vi "Charging_Wait for Charge State.vi"(6 "2nd expected ChargingState (NaN)":string="NaN", 7 "expected ChargingState":string="CHARGE_CC_SLOW-3", 8 "error in":errorcluster, 9 "Abort Threshold (42 C)":dbl=42.0 format="%5.5f", 10 "Critical Threshold (41 C)":dbl=41.0 format="%5.5f", 11 "Warning Threshold (40 C)":dbl=40.0 format="%5.5f") -> (0 "error out":errorcluster, 1 "Transition Interval":dbl[unit]=nan caption="elapsed time" format="%.1f", 2 "IPG Temperature (C)":dbl=nan caption="IPG temperature" format="%.1f", 3 "actual ChargingState":string, 4 "IPG_ReceivedLevel":dbl=nan, 5 "TemperatureLevel":dbl=nan)   [LabVIEW 2010]
doc: "This function polls the IPG temperature and charge status until the expected charging state, IPG temperature limit, time-out, or an error occurs. A Stopwatch popup displays the elapsed time while polling occurs.\n\nCharging States:\nCHARGE_OFF-0\nCHARGE_PRE_CONDITION-1\nCHARGE_CC_FAST-2\nCHARGE_CC_SLOW-3\nCHARGE_COMPLETE-4\nCHARGE_ERROR-5"
panel:
  out "IPG":dbl(slide) scale=37.0..43.0
  in  "temperature limit (43 C)":dbl=43.0 caption="Time Target (s)" format="%.1f"
  out "temperature exceeded":bool
  out "expected charge state":bool
  out "timeout exceeded":bool
  out "done":bool
  in  "timeout (180s)":dbl[unit]=180.0 caption="Time Target (s)" format="%.1f"
  # "GEN CALS"
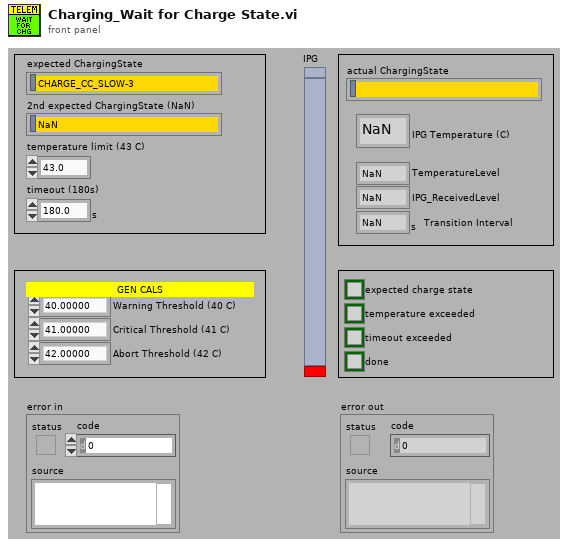
[diagram p1: front panel]
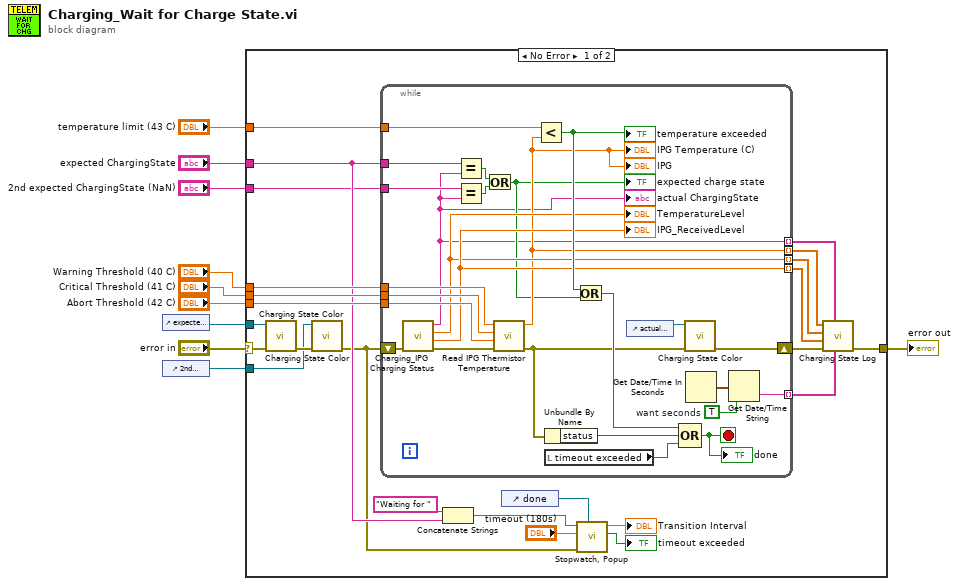
[diagram p0: block diagram]
diagram:
  n1 = control-ref of="expected ChargingState"() -> (w3:refnum<vi>)
  n2 = control-ref of="2nd expected ChargingState (NaN)"() -> (w1:refnum<vi>)
  n3 = case shown="No Error" "error in" {
    selector: "error in" -> [w16 w61]
    tunnel: [w22 w61] -> w10
    tunnel: "temperature limit (43 C)" -> [w31 _]
    tunnel: "expected ChargingState" -> [w25 _]
    tunnel: "Abort Threshold (42 C)" -> [w30 _]
    tunnel: "Critical Threshold (41 C)" -> [w29 _]
    tunnel: "Warning Threshold (40 C)" -> [w28 _]
    tunnel: w3 -> [w15 _]
    tunnel: "2nd expected ChargingState (NaN)" -> [w14 _]
    tunnel: w1 -> [w11 _]
    frame No Error {
      n4 = call "Charging State Color.vi"("error in"=w16, "Str Refnum"=w15) -> ("error out"=w13:errorcluster)  [unwired: 5 in]
      n5 = call "Charging State Color.vi"("error in"=w13, "Str Refnum"=w11) -> ("error out"=w12:errorcluster)  [unwired: 5 in]
      n6 = while {
        shift-right: [w44] -> w23
        shift-left: w12 -> [w37]
        tunnel: w31 -> [w60]
        tunnel: w25 -> [w59]
        tunnel: w30 -> [w58]
        tunnel: w29 -> [w57]
        tunnel: w28 -> [w56]
        tunnel: [w50] -> w21 mode=indexing
        tunnel: [w48] -> w20 mode=indexing
        tunnel: [w47] -> w19 mode=indexing
        tunnel: [w38] -> w18 mode=indexing
        tunnel: [w45] -> w17 mode=indexing
        tunnel: w14 -> [w42]
        stop <- w49 stop-if-true
        w46 = TRUE  # want seconds
        n7 = call "Charging_IPG Charging Status.vi"("error in"=w37) -> ("error out"=w36:errorcluster, "IPG_ReceivedLevel"=w48:dbl, "TemperatureLevel"=w47:dbl, "ChargingState"=w38:string)  [unwired: 7 in]
        "actual ChargingState" <- w38
        "TemperatureLevel" <- w47
        "IPG_ReceivedLevel" <- w48
        n8 = Equal?(x=w59, y=w38) -> (x = y?=w41:bool)
        n9 = Equal?(x=w42, y=w38) -> (x = y?=w40:bool)
        n10 = Or(x=w41, y=w40) -> (x .or. y?=w39:bool)
        "expected charge state" <- w39
        n11 = call "Read IPG Thermistor Temperature.vi"("error in"=w36, "Abort Threshold (42 C)"=w58, "Critical Threshold (41 C)"=w57, "Warning Threshold (40 C)"=w56) -> ("error out"=w35:errorcluster, "Compensated Temperature (C)"=w45:dbl)  [unwired: 4 in, 2 out]
        "IPG Temperature (C)" <- w45
        "IPG" <- w45
        n12 = Less?(x=w60, y=w45) -> (x < y?=w55:bool)
        "temperature exceeded" <- w55
        n13 = Unbundle By Name(w35) -> ("status"=w54:bool)
        n14 = local read "timeout exceeded"() -> (w52:bool)
        n15 = Or(x=w55, y=w39) -> (x .or. y?=w53:bool)
        n16 = control-ref of="actual ChargingState"() -> (w43:refnum<vi>)
        n17 = Compound Arithmetic op=OR(w53, w54, w52) -> (w49:bool)
        "done" <- w49
        n18 = call "Charging State Color.vi"("error in"=w35, "Str Refnum"=w43) -> ("error out"=w44:errorcluster)  [unwired: 5 in]
        n19 = Get Date/Time In Seconds() -> (seconds since 1Jan1904=w51:timestamp)
        n20 = Get Date/Time String(seconds (now)=w51, want seconds? (F)=w46) -> (time string=w50:string)  [unwired: 1 in, 1 out]
      }
      n21 = Concatenate Strings("Waiting for " ("Front Panel Window:Title"), w25) -> (w24:string)
      n22 = control-ref of="done"() -> (w33:refnum<vi>)
      n23 = call "Stopwatch, Popup.vi"("Stop (Bool) Refnum"=w33, "error in (no error)"=w12, "Time Target"="timeout (180s)", "Front Panel Window:Title"=w24) -> ("Time has Elapsed"=→"timeout exceeded":bool, "Elapsed Time (Knob)"=→"Transition Interval":dbl[unit])  [unwired: 5 in, 1 out]
      n24 = call "Charging State Log.vi"("Timestamp"=w21, "Charging State"=w18, "error in"=w23, "Rcvd Level"=w20, "Temp Level"=w19, "IPG Temp"=w17) -> ("error out"=w22:errorcluster)  [unwired: 5 in]
    }
    frame Error {
    }
  }
  "error out" <- w10
